vi "action.vi"(0 "HGF_SVVisitor_runMon in":refnum<class "HGF_SVMonitorVisitor.lvclass">, 2 "HGF_Visitable":refnum<class "HGF_Visitable.lvclass">, 5 "error in (no error)":errorcluster) -> (14 "HGF_SVVisitor_runMon out":refnum<class "HGF_SVMonitorVisitor.lvclass">, 16 "dup HGF_Visitable":refnum<class "HGF_Visitable.lvclass">, 19 "error out":errorcluster)   [LabVIEW 2012, in "HGF_SV.lvlib" / "HGF_SVMonitorVisitor.lvclass"]
doc: "This is a dynamic dispatch VI that is called from Visitor.visit(). It will call member VIs of Visitable to perform the requested action which means: calling public methods of Visitable child class.\n\n<B>Hint:</B> This method is abstract and need to be implemented by child classes."
uses:
  HGF_SVMonitorVisitor.lvclass
  HGF_BaseClasses/HGF_Visitable/HGF_Visitable.lvclass
  HGF_Monitor/HGF_Monitor.lvclass
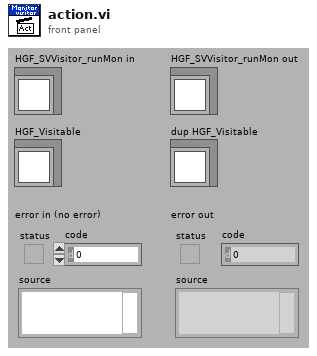
[diagram p1: front panel]
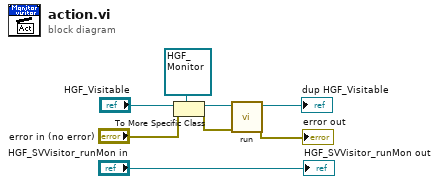
[diagram p0: block diagram]
diagram:
  n1 = To More Specific Class(target class=refnum<class "HGF_Monitor.lvclass"> refnum ("HGF_SV.lvlib:HGF_Monitor.lvclass"), reference="HGF_Visitable", error in="error in (no error)") -> (specific class reference=w6:refnum<class "HGF_Monitor.lvclass">, error out=w4:errorcluster)
  n2 = call-dynamic "run.vi"("error in (no error)"=w4, "HGF_Monitor in"=w6) -> ("error out"=→"error out":errorcluster, "HGF_Monitor out"=→"dup HGF_Visitable":refnum<class "HGF_Monitor.lvclass">)  [unwired: 8 in]
  "HGF_SVVisitor_runMon out" <- "HGF_SVVisitor_runMon in"
